vi "ConstructDataValue.vi"(4 "label":bool, 5 "value":bool, 8 "Value":variant, 9 "module namespace":string="lvDT.") -> (1 "type":string, 3 "value":string)   [LabVIEW 2014, in "Raspberry Pi Compatible Compiler for LabVIEW.lvlib" / "Python Functions.lvlib"]
uses:
  Parsing/Python Functions.lvlib
  <vilib>/Utility/VariantDataType/Type.ctl
  <vilib>/Utility/VariantDataType/RefnumType.ctl
  <vilib>/Utility/VariantDataType/VariantType.lvlib
  Raspberry Pi Compatible Compiler for LabVIEW.lvlib
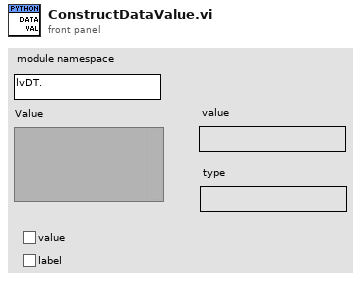
[diagram p1: front panel]
types:
  T1 = typedef "VariantType.lvlib/RefnumType.ctl" = enum16{"NotARefnum", "UnknownRefnum", "Generic", "Datalog", "ByteStream", "Device", "Occurence", "TCPNetConnection", "Auto", "Menu", "Imaq", "Hardware", "DataSocket", "Visa", "IVI", "UDPNetConnection", "Notifier", "Queue", "Irda", "EventReg", "DotNet", "UserEvent", "Callback", "UNUSED_EMPTY_POSITION", "BlueToothNetConnection", "LVObjApp", "LVObjVI", "LVObjUnknown", "GenericClass", "UserDefinedRefnumTag", "DataValue", "RT FIFO", "TDMS File"}
  T2 = typedef "VariantType.lvlib/Type.ctl" = enum8{"Invalid Type", "Void", "I8", "I16", "I32", "I64", "U8", "U16", "U32", "U64", "Single Float", "Double Float", "Extended Float", "Single Complex", "Double Complex", "Extended Complex", "Enum U8", "Enum U16", "Enum U32", "Enum U64", "Single Float With Unit", "Double Float With Unit", "Extended Float With Unit", "Single Complex with Unit", "Double Complex with Unit", "Extended Complex with Unit", "Boolean", "String", "Path", "Picture", "Tag", "Array", "Cluster", "Variant", "LV Variant", "Waveform", "Timestamp", "Digital Waveform", "Digital Data", "ExpressData", "Refnum", "External Data", "VI", "Poly VI", "LabVIEW Class Instance", "Fixed Point"}
  T3 = typedef "VariantType.lvlib/MemoryInfo.ctl" = cluster{"Type":T4, "Size":u32}
  T4 = typedef "VariantType.lvlib/MemoryType.ctl" = enum16{"Variable", "Fixed", "Bounded"}
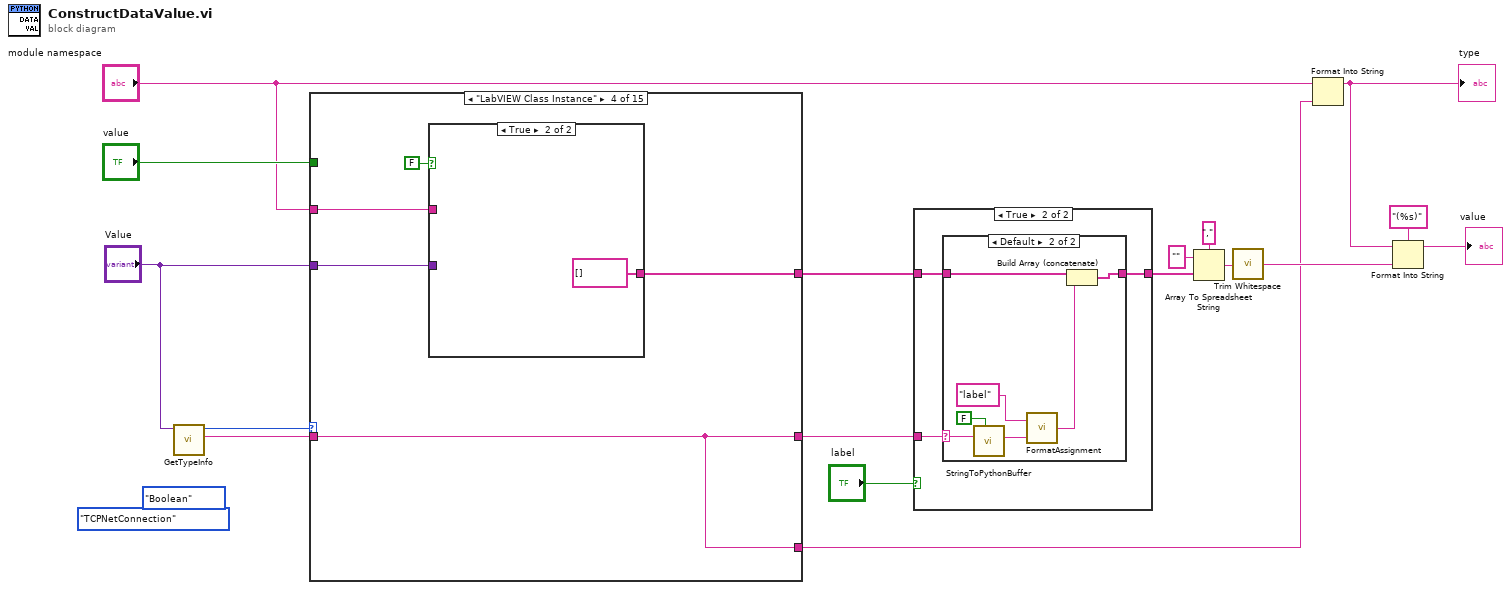
[diagram p0: block diagram]
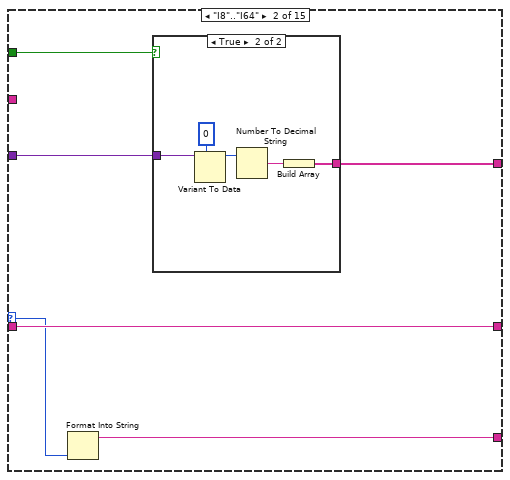
[diagram p5: hidden frame]
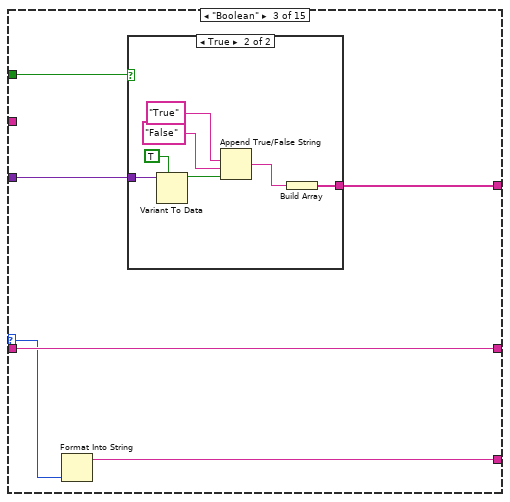
[diagram p7: hidden frame]
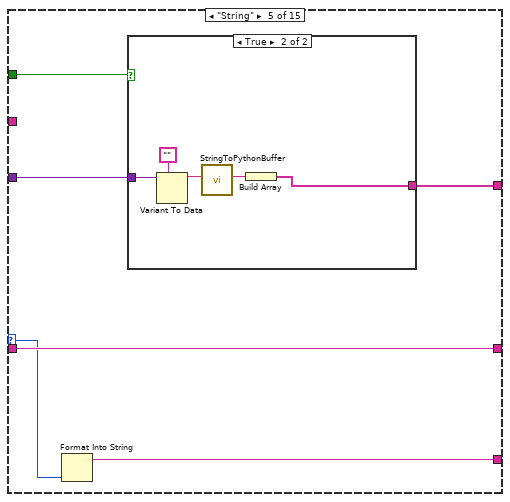
[diagram p10: hidden frame]
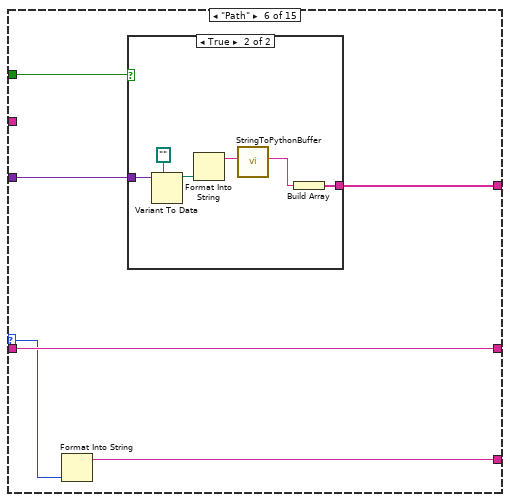
[diagram p12: hidden frame]
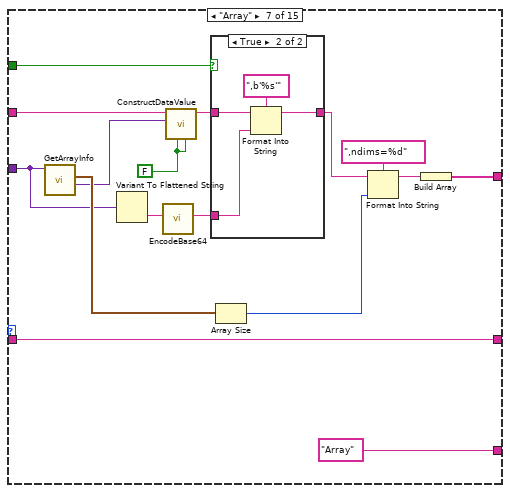
[diagram p14: hidden frame]
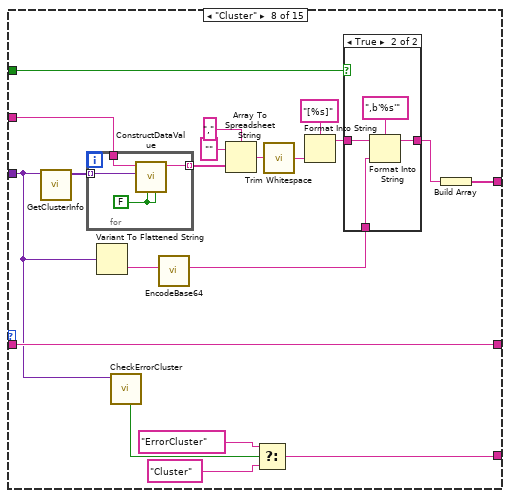
[diagram p16: hidden frame]
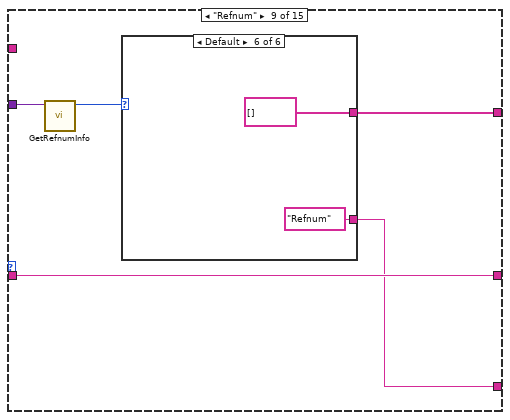
[diagram p18: hidden frame]
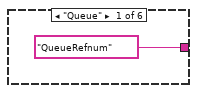
[diagram p19: hidden frame]
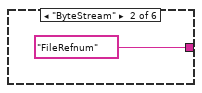
[diagram p20: hidden frame]
diagram:
  (unwired) RefnumType."TCPNetConnection" ("ReferenceType")
  (unwired) Type."Boolean" ("Type Enum")
  n1 = call <vilib>:"GetTypeInfo.vi"("Variant"="Value") -> ("Name"=w15:string, "Type Enum"=w17:T2)  [unwired: 6 in, 3 out]
  n2 = case shown="\"LabVIEW Class Instance\"" w17 {
    selector: w17 -> [_ w21 w33 _ w52 w63 _ _ _ w141 w156 _ _ _ w194]
    tunnel: "Value" -> [_ w24 w31 w47 w50 w61 w82 w97 w126 w143 w157 w164 w175 w186 w198]
    tunnel: "module namespace" -> [_ _ _ w45 _ _ w84 w111 _ _ _ _ _ _ _]
    tunnel: [_ w23 w30 w46 w49 w60 w72 w98 w124 w134 w149 w161 w172 w183 w196] -> w4
    tunnel: w15 -> [w18 w22 w35 w43 w54 w65 w85 w106 w123 w140 w155 w162 w173 w184 w197]
    tunnel: [w18 w22 w35 w43 w54 w65 w85 w106 w123 w140 w155 w162 w173 w184 w197] -> w14
    tunnel: [_ w20 w34 w43 w53 w64 "Array" w94 w122 w142 w146 "SGL" "DBL" "EXT" w193] -> w2
    tunnel: "value" -> [_ w19 w32 _ w51 w62 w79 w102 _ w138 w153 w160 w171 w182 w195]
    frame Default {
    }
    frame "I8".."I64" {
      n3 = Format Into String(w21) -> (resulting string=w20:string)  [unwired: 3 in, 1 out]
      n4 = case shown="True" w19 {
        tunnel: w24 -> [_ w28]
        tunnel: [_ w25] -> w23
        frame False {
        }
        frame True {
          n5 = Variant To Data(type=i64 0, Variant=w28) -> (data=w27:i64)  [unwired: 1 in, 1 out]
          n6 = Number To Decimal String(number=w27) -> (decimal integer string=w26:string)  [unwired: 1 in]
          n7 = Build Array(w26) -> (w25:string[])
        }
      }
    }
    frame "Boolean" {
      n8 = Format Into String(w33) -> (resulting string=w34:string)  [unwired: 3 in, 1 out]
      n9 = case shown="True" w32 {
        tunnel: w31 -> [_ w42]
        tunnel: [_ w40] -> w30
        frame False {
        }
        frame True {
          n10 = Variant To Data(type=TRUE, Variant=w42) -> (data=w39:bool)  [unwired: 1 in, 1 out]
          n11 = Append True/False String(1:w39, 2:"False" ("true string"), 3:"True" ("true string")) -> (0:w38:string)  [unwired: 1 in]
          n12 = Build Array(w38) -> (w40:string[])
        }
      }
    }
    frame "LabVIEW Class Instance" {
      n13 = case shown="True" FALSE {
        tunnel: w47 -> [_ _]
        tunnel: [_ string[] []] -> w46
        tunnel: w45 -> [_ _]
        frame False {
        }
        frame True {
        }
      }
    }
    frame "String" {
      n14 = Format Into String(w52) -> (resulting string=w53:string)  [unwired: 3 in, 1 out]
      n15 = case shown="True" w51 {
        tunnel: w50 -> [_ w59]
        tunnel: [_ w58] -> w49
        frame False {
        }
        frame True {
          n16 = Variant To Data(type="", Variant=w59) -> (data=w56:string)  [unwired: 1 in, 1 out]
          n17 = call "StringToPythonBuffer.vi"("string"=w56) -> ("python string"=w55:string)  [unwired: 8 in]
          n18 = Build Array(w55) -> (w58:string[])
        }
      }
    }
    frame "Path" {
      n19 = Format Into String(w63) -> (resulting string=w64:string)  [unwired: 3 in, 1 out]
      n20 = case shown="True" w62 {
        tunnel: w61 -> [_ w71]
        tunnel: [_ w70] -> w60
        frame False {
        }
        frame True {
          n21 = Variant To Data(type=path "", Variant=w71) -> (data=w68:path)  [unwired: 1 in, 1 out]
          n22 = Format Into String(w68) -> (resulting string=w67:string)  [unwired: 3 in, 1 out]
          n23 = call "StringToPythonBuffer.vi"("string"=w67) -> ("python string"=w66:string)  [unwired: 8 in]
          n24 = Build Array(w66) -> (w70:string[])
        }
      }
    }
    frame "Array" {
      w81 = FALSE ("label")
      n25 = call <vilib>:"GetArrayInfo.vi"("Variant"=w82) -> ("ArrayElement"=w83:variant, "Array Lengths"=w87:T3[])  [unwired: 7 in, 2 out]
      n26 = Variant To Flattened String(Variant=w82) -> (data string=w86:string)  [unwired: 1 out]
      n27 = call "EncodeBase64.vi"("string"=w86) -> ("base64 string"=w77:string)  [unwired: 10 in]
      n28 = call "ConstructDataValue.vi"("label"=w81, "value"=w81, "Value"=w83, "module namespace"=w84) -> ("value"=w78:string)  [unwired: 4 in, 1 out]
      n29 = case shown="True" w79 {
        tunnel: w78 -> [w88 w92]
        tunnel: w77 -> [_ w89]
        tunnel: [w88 w90] -> w73
        frame False {
        }
        frame True {
          n30 = Format Into String(format string=",b'%s'", initial string=w92, w89) -> (resulting string=w90:string)  [unwired: 1 in, 1 out]
        }
      }
      n31 = Array Size(array=w87) -> (size(s)=w75:i32)
      n32 = Format Into String(format string=",ndims=%d", initial string=w73, w75) -> (resulting string=w74:string)  [unwired: 1 in, 1 out]
      n33 = Build Array(w74) -> (w72:string[])
    }
    frame "Cluster" {
      n34 = call <vilib>:"GetClusterInfo.vi"("Variant"=w97) -> ("Cluster Elements"=w112:variant[])  [unwired: 9 in, 1 out]
      n35 = for {
        tunnel: w112 -> [w121] mode=indexing
        tunnel: w111 -> [w120]
        tunnel: [w119] -> w110 mode=indexing
        w118 = FALSE ("value")
        n36 = call "ConstructDataValue.vi"("label"=w118, "value"=w118, "Value"=w121, "module namespace"=w120) -> ("value"=w119:string)  [unwired: 4 in, 1 out]
      }
      n37 = Variant To Flattened String(Variant=w97) -> (data string=w105:string)  [unwired: 1 out]
      n38 = call "CheckErrorCluster.vi"("Value"=w97) -> ("error cluster"=w96:bool)  [unwired: 8 in]
      n39 = call "EncodeBase64.vi"("string"=w105) -> ("base64 string"=w100:string)  [unwired: 10 in]
      n40 = Array To Spreadsheet String(delimiter (Tab)=",", array=w110, 3:"" ("format string")) -> (spreadsheet string=w107:string)
      n41 = Select(t="ErrorCluster", s=w96, f="Cluster") -> (s? t:f=w94:string)
      n42 = call <vilib>:"Trim Whitespace.vi"("string"=w107) -> ("trimmed string"=w104:string)  [unwired: 1 in]
      n43 = Format Into String(format string="[%s]", w104) -> (resulting string=w101:string)  [unwired: 2 in, 1 out]
      n44 = case shown="True" w102 {
        tunnel: w101 -> [w113 w116]
        tunnel: [w113 w115] -> w99
        tunnel: w100 -> [_ w114]
        frame False {
        }
        frame True {
          n45 = Format Into String(format string=",b'%s'", initial string=w116, w114) -> (resulting string=w115:string)  [unwired: 1 in, 1 out]
        }
      }
      n46 = Build Array(w99) -> (w98:string[])
    }
    frame "Refnum" {
      n47 = call <vilib>:"GetRefnumInfo.vi"("Variant"=w126) -> ("ReferenceType"=w125:T1)  [unwired: 7 in, 3 out]
      n48 = case shown="Default" w125 {
        tunnel: [_ _ _ _ _ string[] []] -> w124
        tunnel: ["QueueRefnum" ("initial string") "FileRefnum" ("initial string") "VisaResource" ("initial string") "TCPRefnum" ("initial string") "UDPRefnum" ("initial string") "Refnum" ("initial string")] -> w122
        frame "Queue" {
        }
        frame "ByteStream" {
        }
        frame "Visa" {
        }
        frame "TCPNetConnection" {
        }
        frame "UDPNetConnection" {
        }
        frame Default {
        }
      }
    }
    frame "U8".."U64" {
      n49 = Not(x=w138) -> (.not. x?=w137:bool)
      n50 = Variant To Data(type=u64 0, Variant=w143) -> (data=w144:u64)  [unwired: 1 in, 1 out]
      n51 = Format Into String(w141) -> (resulting string=w142:string)  [unwired: 3 in, 1 out]
      n52 = Number To Decimal String(number=w144) -> (decimal integer string=w139:string)  [unwired: 1 in]
      n53 = Swap Values(12:"", 13:w137, 14:w139) -> (3:w135:string)  [unwired: 1 out]
      n54 = Build Array(w135) -> (w134:string[])
    }
    frame "Enum U8".."Enum U64" {
      n55 = Not(x=w153) -> (.not. x?=w152:bool)
      n56 = Variant To Data(type=u64 0, Variant=w157) -> (data=w158:u64)  [unwired: 1 in, 1 out]
      n57 = Format Into String(w156) -> (resulting string=w148:string)  [unwired: 3 in, 1 out]
      n58 = Number To Decimal String(number=w158) -> (decimal integer string=w154:string)  [unwired: 1 in]
      n59 = Swap Values(12:"", 13:w152, 14:w154) -> (3:w150:string)  [unwired: 1 out]
      n60 = Match Pattern(string=w148, regular expression="Enum ") -> (after substring=w146:string)  [unwired: 1 in, 3 out]
      n61 = Build Array(w150) -> (w149:string[])
    }
    frame "Single Float" {
      n62 = case shown="True" w160 {
        tunnel: w164 -> [_ w169]
        tunnel: [_ w165] -> w161
        frame False {
        }
        frame True {
          n63 = Variant To Flattened String(Variant=w169) -> (data string=w170:string)  [unwired: 1 out]
          n64 = call "EncodeBase64.vi"("string"=w170) -> ("base64 string"=w167:string)  [unwired: 10 in]
          n65 = Format Into String(format string="b'%s'", w167) -> (resulting string=w166:string)  [unwired: 2 in, 1 out]
          n66 = Build Array(w166) -> (w165:string[])
        }
      }
    }
    frame "Double Float" {
      n67 = case shown="True" w171 {
        tunnel: w175 -> [_ w180]
        tunnel: [_ w176] -> w172
        frame False {
        }
        frame True {
          n68 = Variant To Flattened String(Variant=w180) -> (data string=w181:string)  [unwired: 1 out]
          n69 = call "EncodeBase64.vi"("string"=w181) -> ("base64 string"=w178:string)  [unwired: 10 in]
          n70 = Format Into String(format string="b'%s'", w178) -> (resulting string=w177:string)  [unwired: 2 in, 1 out]
          n71 = Build Array(w177) -> (w176:string[])
        }
      }
    }
    frame "Extended Float" {
      n72 = case shown="True" w182 {
        tunnel: w186 -> [_ w191]
        tunnel: [_ w187] -> w183
        frame False {
        }
        frame True {
          n73 = Variant To Flattened String(Variant=w191) -> (data string=w192:string)  [unwired: 1 out]
          n74 = call "EncodeBase64.vi"("string"=w192) -> ("base64 string"=w189:string)  [unwired: 10 in]
          n75 = Format Into String(format string="b'%s'", w189) -> (resulting string=w188:string)  [unwired: 2 in, 1 out]
          n76 = Build Array(w188) -> (w187:string[])
        }
      }
    }
    frame "Timestamp" {
      n77 = Format Into String(w194) -> (resulting string=w193:string)  [unwired: 3 in, 1 out]
      n78 = case shown="True" w195 {
        tunnel: w198 -> [_ w203]
        tunnel: [_ w199] -> w196
        frame False {
        }
        frame True {
          n79 = Variant To Flattened String(Variant=w203) -> (data string=w204:string)  [unwired: 1 out]
          n80 = call "EncodeBase64.vi"("string"=w204) -> ("base64 string"=w201:string)  [unwired: 10 in]
          n81 = Format Into String(format string="b'%s'", w201) -> (resulting string=w200:string)  [unwired: 2 in, 1 out]
          n82 = Build Array(w200) -> (w199:string[])
        }
      }
    }
  }
  n83 = case shown="True" "label" {
    tunnel: w14 -> [_ w206]
    tunnel: w4 -> [w205 w208]
    tunnel: [w205 w207] -> w12
    frame False {
    }
    frame True {
      n84 = case shown="Default" w206 {
        selector: w206 -> [_ w211]
        tunnel: w208 -> [w209 w216]
        tunnel: [w209 w215] -> w207
        frame "" {
        }
        frame Default {
          n85 = call "StringToPythonBuffer.vi"("Buffer"=FALSE, "string"=w211) -> ("python string"=w212:string)  [unwired: 7 in]
          n86 = call "FormatAssignment.vi"("value"=w212, "name"="label") -> ("python assignment"=w214:string)
          n87 = Build Array (concatenate)(w216, w214) -> (w215:string[])
        }
      }
    }
  }
  n88 = Array To Spreadsheet String(delimiter (Tab)=",", array=w12, 3:"" ("format string")) -> (spreadsheet string=w10:string)
  n89 = call <vilib>:"Trim Whitespace.vi"("string"=w10) -> ("trimmed string"=w8:string)  [unwired: 1 in]
  n90 = Format Into String(initial string="module namespace", w2) -> (resulting string=w1:string)  [unwired: 2 in, 1 out]
  "type" <- w1
  n91 = Format Into String(format string="(%s)", initial string=w1, w8) -> (resulting string=→"value":string)  [unwired: 1 in, 1 out]
